vi "Scheduling_gif.vi"   [LabVIEW 2020, in "CIRCUS_uServices.lvlib" / "Scheduler.lvlib" / "Scheduler.lvclass"]
uses:
  Scheduler.lvclass
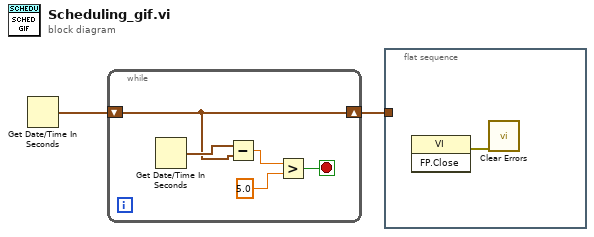
[diagram p0: block diagram]
diagram:
  n1 = Get Date/Time In Seconds() -> (seconds since 1Jan1904=w2:timestamp)
  n2 = while {
    shift-right: [w3] -> w1
    shift-left: w2 -> [w3]
    stop <- w5 stop-if-true
    n3 = Get Date/Time In Seconds() -> (seconds since 1Jan1904=w4:timestamp)
    n4 = Subtract(x=w4, y=w3) -> (x-y=w7:dbl)
    n5 = Greater?(x=w7, y=5.0) -> (0:w5:bool)
  }
  n6 = flat-sequence {
    tunnel: w1 -> [_]
    frame #0 {
      n7 = invoke class="VI" method="FP.Close"() -> (error out=w8:errorcluster)  [unwired: 3 in, 2 out]
      n8 = call <vilib>:"Clear Errors.vi"("error in (no error)"=w8) -> ()  [unwired: 5 in, 2 out]
    }
  }
